vi "ex_WriteExcelData.vi"(0 "file path":path, 1 "Signals":waveform(dbl)[](array[waveform]), 2 "Excel refnum":T1, 3 "absolulte time (yes:T)":bool=TRUE, 4 "overwrite_mode_multi":T2(ring)=enum."overwrite & backup", 5 "overwrite_mode":T3(ring)=enum."overwrite & backup", 6 "x_columns":u16(ring) items=["None", "One", "Multiple"], 7 "error in (no error)":errorcluster, 8 "file dialog?":bool, 9 "Flush":bool, 11 "timestamp format":string, 12 "multi_file":bool, 14 "new file?":bool) -> (17 "operator cancelled?":bool, 20 "file path out":path, 22 "Excel refnum out":T1, 27 "error out":errorcluster)   [LabVIEW 2020]
uses:
  <vilib>/express/express shared/NI_ExcelFile/Ctrls/ExcelRefnum.ctl
  <vilib>/express/express shared/NI_ExcelFile/Ctrls/MainData.ctl
  <vilib>/express/express shared/NI_ExcelFile/Ctrls/StreamMode.ctl
  <vilib>/express/express shared/NI_ExcelFile/Ctrls/TimeColumnMode.ctl
  <vilib>/express/express shared/NI_ExcelFile/Ctrls/FileAttribute.ctl
  <vilib>/express/express shared/NI_ExcelFile/Ctrls/Columns.ctl
  <vilib>/express/express shared/NI_ExcelFile/Ctrls/ColumnInfo.ctl
  <vilib>/express/express shared/NI_ExcelFile/Ctrls/DataType.ctl
  <vilib>/express/express shared/NI_ExcelFile/Ctrls/wd_recordInfo.ctl
  <vilib>/express/express shared/NI_ExcelFile/Ctrls/disk_TemplateFile.ctl
  <vilib>/express/express shared/NI_ExcelFile/Ctrls/meta_file.ctl
  <vilib>/express/express shared/NI_ExcelFile/Ctrls/meta_Block.ctl
  <vilib>/express/express shared/NI_ExcelFile/Ctrls/meta_BlockType.ctl
  <vilib>/express/express shared/NI_ExcelFile/Ctrls/FileOperation.ctl
  <vilib>/express/express shared/ExFile.llb/ex_FileGlobals.vi
  <vilib>/express/express shared/NI_ExcelFile/SubVIs/WriteData (WFM).vi
  <vilib>/express/express shared/NI_ExcelFile/NI_ExcelFile.lvlib
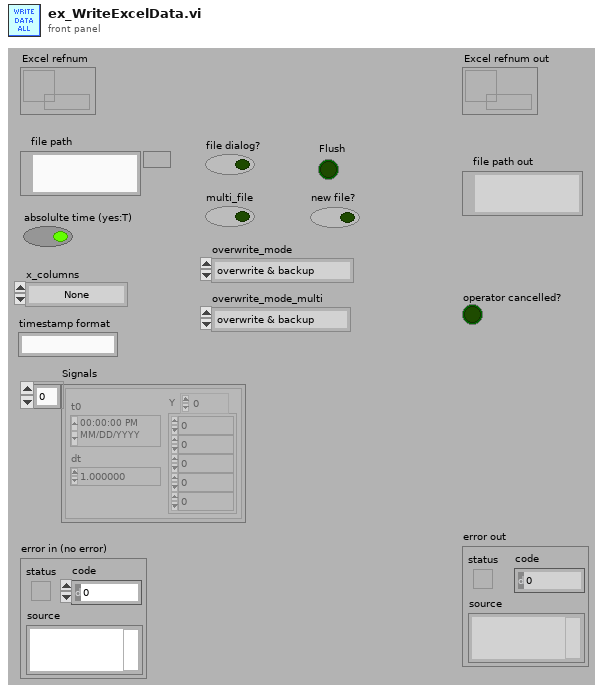
[diagram p1: front panel]
types:
  T1 = typedef "NI_ExcelFile.lvlib/ExcelRefnum.ctl" = refnum<data-value>
  T2 = enum16{"overwrite", "overwrite & backup", "next avail"}
  T3 = enum16{"overwrite", "overwrite & backup", "append", "next avail"}
  T4 = enum16{"Append values", "Create", "Replace values at index", "Replace all values"}
  T5 = typedef "NI_ExcelFile.lvlib/TimeColumnMode.ctl" = enum16{"Empty", "OnePerCh", "One"}
  T6 = typedef "NI_ExcelFile.lvlib/FileOperation.ctl" = enum16{"open or create", "open", "create or replace", "create"}
  T7 = enum16{"existing file", "new file", "new or existing file", "existing dir", "new dir", "new or existing dir", "existing file (use LLBs)", "new file (use LLBs)", "new or existing file (use LLBs)", "new or existing file or directory (use LLBs)"}
  T8 = cluster{"message":string, "T button name":string, "F button name":string}
  T9 = cluster{"Start Timestamp":timestamp, "Timestamp":timestamp, "Relative Time?":bool, "X Dimension":string, "Signal Name":string, "Y Units":string, "X0":timestamp, "dX":dbl, "nPoints":i32}[]
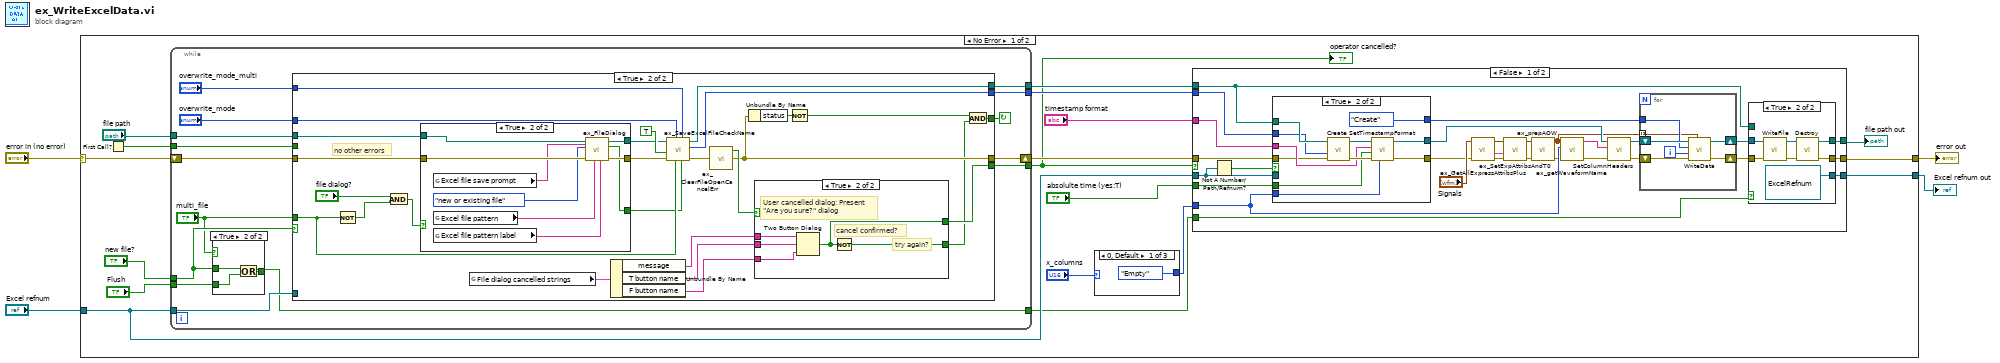
[diagram p0: block diagram]
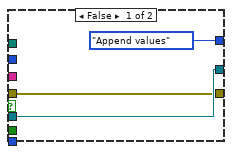
[diagram p3: hidden frame]
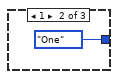
[diagram p5: hidden frame]
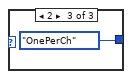
[diagram p6: hidden frame]
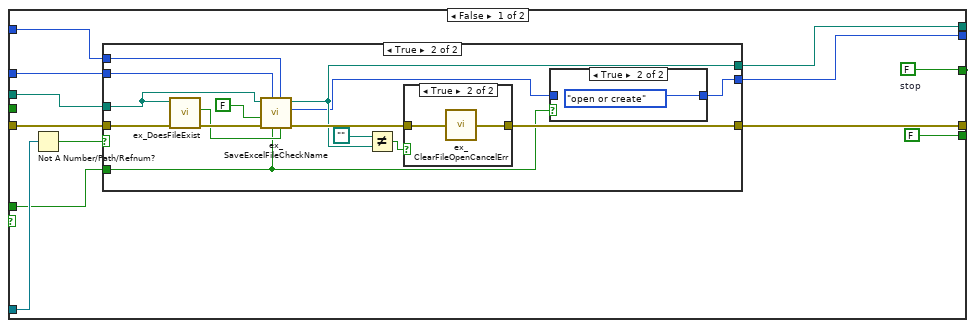
[diagram p8: hidden frame]
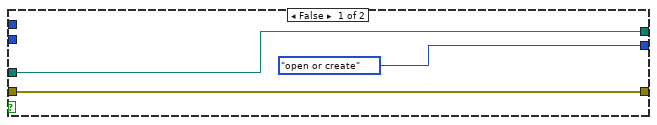
[diagram p9: hidden frame]
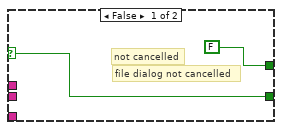
[diagram p12: hidden frame]
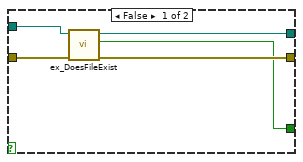
[diagram p13: hidden frame]
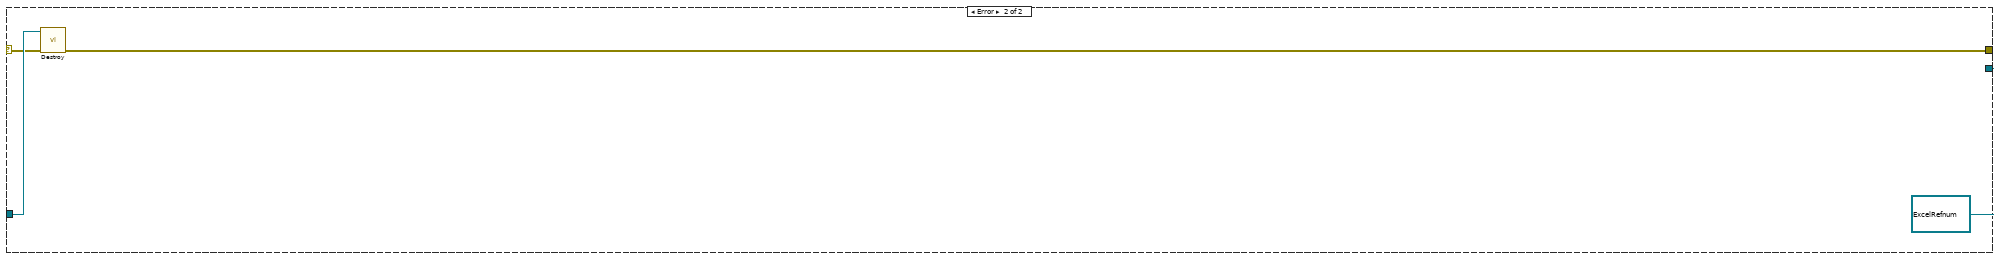
[diagram p14: hidden frame]
diagram:
  n1 = case shown="No Error" "error in (no error)" {
    selector: "error in (no error)" -> [w22 w192]
    tunnel: [w10 w191] -> w1
    tunnel: "Excel refnum" -> [w6 w193]
    tunnel: [w7 T1 refnum ("Excel refnum")] -> w2
    frame No Error {
      n2 = First Call?() -> (First Call?: T/F=w20:bool)
      n3 = while {
        tunnel: "new file?" -> [w97]
        tunnel: "file path" -> [w102]
        tunnel: w20 -> [w98]
        tunnel: "Flush" -> [w96]
        shift-right: [w93] -> w11
        shift-left: w22 -> [w103]
        tunnel: [w92] -> w13
        tunnel: [w91] -> w12
        tunnel: [w90] -> w8
        tunnel: w6 -> [w94]
        tunnel: [w89] -> w5
        stop <- w101 continue-if-true
        n4 = case shown="True" "multi_file" {
          tunnel: w97 -> [_ w107]
          tunnel: w96 -> [w104 w106]
          tunnel: [w104 w105] -> w89
          frame False {
          }
          frame True {
            n5 = Or(x=w107, y=w106) -> (x .or. y?=w105:bool)
          }
        }
        n6 = case shown="True" w97 {
          tunnel: w103 -> [w116 w145]
          tunnel: w102 -> [w118 w161]
          tunnel: [w117 w147] -> w93
          tunnel: [w119 w152] -> w101
          tunnel: "overwrite_mode_multi" -> [w114 w166]
          tunnel: "overwrite_mode" -> [w115 w167]
          tunnel: "multi_file" -> [w109 w163]
          tunnel: w98 -> [_ _]
          tunnel: [w108 w149] -> w91
          tunnel: [w113 w150] -> w92
          tunnel: [FALSE ("T button?") w146] -> w90
          tunnel: w94 -> [w111 _]
          frame False {
            w119 = FALSE  # stop
            n7 = Not A Number/Path/Refnum?(number/path/refnum=w111) -> (NaN/Path/Refnum?=w110:bool)
            n8 = case shown="True" w110 {
              tunnel: w118 -> [w121 w133]
              tunnel: w116 -> [w122 w136]
              tunnel: [w122 w137] -> w117
              tunnel: w115 -> [_ w130]
              tunnel: w114 -> [_ w129]
              tunnel: w109 -> [_ w125]
              tunnel: [w121 w126] -> w113
              tunnel: [FileOperation."open or create" ("function") w123] -> w108
              frame False {
              }
              frame True {
                n9 = call <vilib>:"ex_DoesFileExist.vi"("error in"=w136, "file path"=w133) -> ("error out"=w131:errorcluster, "file exists"=w128:bool)  [unwired: 4 out]
                n10 = call <vilib>:"ex_SaveExcelFileCheckName.vi"("file exists?"=w128, "overwrite_mode_multi"=w129, "multi_file"=w125, "overwrite_mode"=w130, "error in (no error)"=w131, "enable file ops"=FALSE, "file path"=w133) -> ("error out"=w127:errorcluster, "function"=w124:T6, "file path out"=w126:path)  [unwired: 2 in]
                n11 = Not Equal?(x=path "", y=w126) -> (x != y?=w134:bool)
                n12 = case shown="True" w134 {
                  tunnel: [w140 w141] -> w137
                  tunnel: w127 -> [w140 w142]
                  frame False {
                  }
                  frame True {
                    n13 = call <vilib>:"ex_ClearFileOpenCancelErr.vi"("error in"=w142) -> ("error out"=w141:errorcluster)  [unwired: 4 out]
                  }
                }
                n14 = case shown="True" w125 {
                  tunnel: [w138 FileOperation."open or create" ("function")] -> w123
                  tunnel: w124 -> [w138 _]
                  frame False {
                  }
                  frame True {
                  }
                }
              }
            }
          }
          frame True {
            # "no other errors"
            n15 = Not(x=w163) -> (.not. x?=w165:bool)
            n16 = And(x="file dialog?", y=w165) -> (x .and. y?=w162:bool)
            n17 = case shown="True" w162 {
              tunnel: w161 -> [w179 w189]
              tunnel: [w178 w188] -> w160
              tunnel: [w177 w187] -> w159
              tunnel: w145 -> [w180 w186]
              tunnel: [w176 w185] -> w158
              frame False {
                n18 = call <vilib>:"ex_DoesFileExist.vi"("error in"=w180, "file path"=w179) -> ("error out"=w177:errorcluster, "file exists"=w176:bool, "dup file path"=w178:path)  [unwired: 3 out]
              }
              frame True {
                n19 = global read "ex_FileGlobals.vi" "Excel file save prompt"() -> (w183:string)
                n20 = global read "ex_FileGlobals.vi" "Excel file pattern"() -> (w181:string)
                n21 = global read "ex_FileGlobals.vi" "Excel file pattern label"() -> (w182:string)
                n22 = call <vilib>:"ex_FileDialog.vi"("pattern label"=w182, "pattern"=w181, "prompt"=w183, "error in (no error)"=w186, "select mode"=T7."new or existing file", "start path"=w189) -> ("error out"=w187:errorcluster, "file exists?"=w185:bool, "selected file path"=w188:path)  [unwired: 3 out]
              }
            }
            n23 = global read "ex_FileGlobals.vi" "File dialog cancelled strings"() -> (w154:T8)
            n24 = Unbundle By Name(w154) -> ("message"=w157:string, "T button name"=w156:string, "F button name"=w155:string)
            n25 = call <vilib>:"ex_SaveExcelFileCheckName.vi"("file exists?"=w158, "overwrite_mode_multi"=w166, "multi_file"=w163, "overwrite_mode"=w167, "error in (no error)"=w159, "enable file ops"=TRUE, "file path"=w160) -> ("error out"=w148:errorcluster, "function"=w149:T6, "file path out"=w150:path)  [unwired: 2 in]
            n26 = call <vilib>:"ex_ClearFileOpenCancelErr.vi"("error in"=w148) -> ("error out"=w147:errorcluster, "cancelled?"=w151:bool)  [unwired: 3 out]
            n27 = Unbundle By Name(w147) -> ("status"=w153:bool)
            n28 = case shown="True" w151 {
              selector: w151 -> [w170 _]
              tunnel: [w170 w174] -> w144
              tunnel: [FALSE ("T button?") w175] -> w146
              tunnel: w155 -> [_ w173]
              tunnel: w157 -> [_ w172]
              tunnel: w156 -> [_ w171]
              frame False {
                # "not cancelled"
                # "file dialog not cancelled"
              }
              frame True {
                # "cancel confirmed?"
                # "try again?"
                # "User cancelled dialog: Present\n\"Are you sure?\" dialog"
                n29 = Two Button Dialog(message=w172, 1:w173, 2:w171) -> (T button?=w175:bool)
                n30 = Not(x=w175) -> (.not. x?=w174:bool)
              }
            }
            n31 = Not(x=w153) -> (.not. x?=w143:bool)
            n32 = And(x=w143, y=w144) -> (x .and. y?=w152:bool)
          }
        }
      }
      "operator cancelled?" <- w8
      n33 = case shown="0, Default" "x_columns" {
        tunnel: [TimeColumnMode."Empty" ("time column mode (0: Empty)") TimeColumnMode."One" ("time column mode (0: Empty)") TimeColumnMode."OnePerCh" ("time column mode (0: Empty)")] -> w14
        frame 0, Default {
        }
        frame 1 {
        }
        frame 2 {
        }
      }
      n34 = case shown="False" w8 {
        tunnel: [w46 w85] -> w7
        tunnel: w14 -> [w38 _]
        tunnel: [w47 w84] -> w10
        tunnel: "absolulte time (yes:T)" -> [w45 _]
        tunnel: "timestamp format" -> [w44 _]
        tunnel: w13 -> [w34 w83]
        tunnel: w12 -> [w37 _]
        tunnel: w11 -> [w36 w84]
        tunnel: [w35 w83] -> w9
        tunnel: w6 -> [w32 w85]
        tunnel: w5 -> [w33 _]
        frame False {
          n35 = Not A Number/Path/Refnum?(number/path/refnum=w32) -> (NaN/Path/Refnum?=w51:bool)
          n36 = case shown="True" w51 {
            tunnel: [w69 w77] -> w27
            tunnel: [w70 w78] -> w42
            tunnel: [T4."Append values" ("operation (0: create)") T4."Create" ("operation (0: create)")] -> w50
            tunnel: w38 -> [_ w79]
            tunnel: w45 -> [_ w76]
            tunnel: w44 -> [_ w75]
            tunnel: w34 -> [_ w74]
            tunnel: w37 -> [_ w73]
            tunnel: w36 -> [w69 w72]
            tunnel: w32 -> [w70 _]
            frame False {
            }
            frame True {
              n37 = call <vilib>:"Create.vi"("error in (no error)"=w72, "operation (0: open or create)"=w73, "file"=w74) -> ("error out"=w80:errorcluster, "Excel refnum out"=w81:T1)  [unwired: 7 in]
              n38 = call <vilib>:"SetTimestampFormat.vi"("time column mode (0: Empty)"=w79, "error in (no error)"=w80, "absolulte time (T)"=w76, "timestamp format"=w75, "Excel refnum"=w81) -> ("error out"=w77:errorcluster, "Excel refnum out"=w78:T1)  [unwired: 5 in]
            }
          }
          n39 = call <vilib>:"ex_GetAllExpressAttribsPlus.vi"("error in"=w27, "Signals in"="Signals") -> ("error out"=w30:errorcluster, "All Express Wave Attributes Plus"=w29:T9, "Signals out"=w31:waveform(dbl)[])  [unwired: 1 in, 6 out]
          n40 = call <vilib>:"ex_SetExpAttribsAndT0.vi"("error in (no error)"=w30, "Express Attributes Plus in"=w29, "Signals"=w31) -> ("error out"=w25:errorcluster, "Signals With Attributes"=w26:waveform(dbl)[])  [unwired: 3 in, 4 out]
          n41 = call <vilib>:"ex_prepAOW.vi"("error in (no error)"=w25, "Dynamic Data"=w26) -> ("error out"=w23:errorcluster, 3:w24:waveform(dbl)[])  [unwired: 1 in, 3 out]
          n42 = call <vilib>:"ex_getWaveformName.vi"("error in (no error)"=w23, "TimeColumnMode"=w38, "Dynamic Data"=w24) -> ("error out"=w40:errorcluster, "WaveName"=w43:string[])  [unwired: 7 in]
          n43 = call <vilib>:"SetColumnHeaders.vi"("error in (no error)"=w40, "column headers"=w43, "Excel refnum"=w42) -> ("error out"=w39:errorcluster, "Excel refnum out"=w41:T1)  [unwired: 7 in]
          n44 = for {
            shift-right: [w68] -> w48
            shift-left: w39 -> [w66]
            shift-right: [w64] -> w49
            shift-left: w41 -> [w67]
            tunnel: w50 -> [w65]
            tunnel: w24 -> [w62] mode=indexing
            i -> [w63]
            n45 = call-poly <vilib>:"WriteData.vi"("WFM"=w62, "error in (no error)"=w66, "channel index (0)"=w63, "operation (0: create)"=w65, "Excel refnum"=w67) -> ("error out"=w68:errorcluster, "Excel refnum out"=w64:T1)  [unwired: 5 in]
          }
          n46 = case shown="True" w33 {
            tunnel: w49 -> [w54 w60]
            tunnel: [w54 T1 refnum ("Excel refnum")] -> w46
            tunnel: [w53 w57] -> w47
            tunnel: w48 -> [w53 w56]
            tunnel: [w52 w55] -> w35
            tunnel: w34 -> [w52 _]
            frame False {
            }
            frame True {
              n47 = call <vilib>:"WriteFile.vi"("error in (no error)"=w56, "Excel refnum"=w60) -> ("error out"=w61:errorcluster, "Excel refnum out"=w59:T1)  [unwired: 8 in]
              n48 = call <vilib>:"Destroy.vi"("error in (no error)"=w61, "Excel refnum"=w59) -> ("error out"=w57:errorcluster, "file path"=w55:path)  [unwired: 8 in]
            }
          }
        }
        frame True {
        }
      }
      "file path out" <- w9
    }
    frame Error {
      n49 = call <vilib>:"Destroy.vi"("error in (no error)"=w192, "Excel refnum"=w193) -> ("error out"=w191:errorcluster)  [unwired: 8 in, 1 out]
    }
  }
  "error out" <- w1
  "Excel refnum out" <- w2
